vi "CalculerPolynome.vi"(6 "Résidu [in]":dbl, 8 "e3 [in]":dbl, 9 "Meilleure poly [in]":dbl[](array[numeric]), 10 "Y":dbl[](array[numeric]), 11 "X":dbl[](array[numeric])) -> (2 "Résidu [out]":dbl, 3 "Meilleur poly [out]":dbl[](array[numeric]))   [LabVIEW 2013]
uses:
  lm64.dll
  lm32.dll
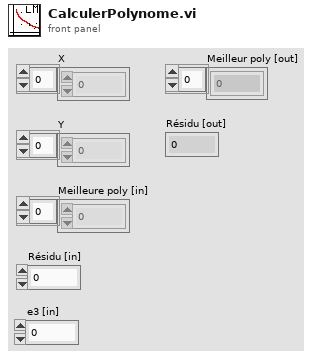
[diagram p1: front panel]
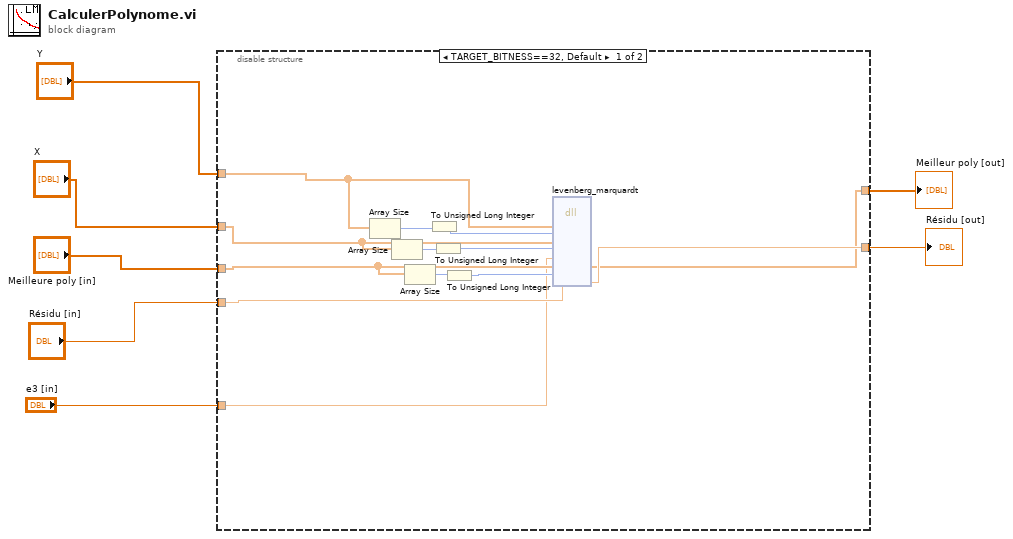
[diagram p0: block diagram]
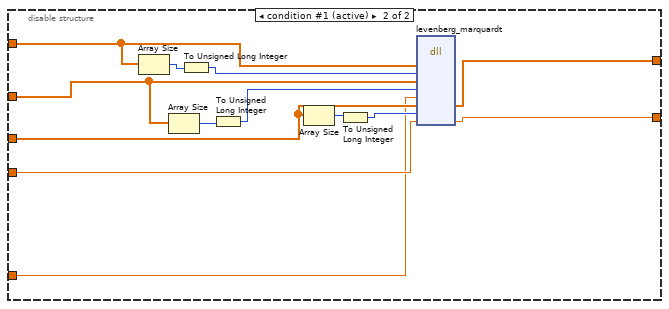
[diagram p2: hidden frame]
diagram:
  n1 = disable-structure shown="TARGET_BITNESS==32, Default" {
    disable-tunnel: "X" -> [w11 w33]
    disable-tunnel: "Y" -> [w14 w32]
    disable-tunnel: "Meilleure poly [in]" -> [w17 w27]
    disable-tunnel: "Résidu [in]" -> [w20 w24]
    disable-tunnel: [w10 w23] -> w6
    disable-tunnel: [w9 w22] -> w7
    disable-tunnel: "e3 [in]" -> [w8 w21]
    frame condition #0 {
      n2 = Array Size(array=w14) -> (size(s)=w15:i32)
      n3 = Array Size(array=w11) -> (size(s)=w12:i32)
      n4 = Array Size(array=w17) -> (size(s)=w18:i32)
      n5 = To Unsigned Long Integer(number=w15) -> (unsigned 32bit integer=w16:u32)
      n6 = To Unsigned Long Integer(number=w12) -> (unsigned 32bit integer=w13:u32)
      n7 = To Unsigned Long Integer(number=w18) -> (unsigned 32bit integer=w19:u32)
      n8 = dll-call lib="C:/Users/Damien/Documents/GitHub/TopView/lm32.dll" fn="levenberg_marquardt"("yobs"=w14, "yobslength"=w16, "xobs"=w11, "xobslength"=w13, "e3"=w8, "polyptr"=w17, "numCoeffs"=w19, "e"=w20) -> ("polyptr"=w9:dbl[], "e"=w10:dbl)  [unwired: 10 in, 2 out]
    }
    frame condition #1 (active) {
      n9 = Array Size(array=w32) -> (size(s)=w29:i32)
      n10 = Array Size(array=w33) -> (size(s)=w31:i32)
      n11 = To Unsigned Long Integer(number=w29) -> (unsigned 32bit integer=w28:u32)
      n12 = To Unsigned Long Integer(number=w31) -> (unsigned 32bit integer=w30:u32)
      n13 = Array Size(array=w27) -> (size(s)=w26:i32)
      n14 = To Unsigned Long Integer(number=w26) -> (unsigned 32bit integer=w25:u32)
      n15 = dll-call lib="C:/Users/Damien/Documents/GitHub/TopView/lm64.dll" fn="levenberg_marquardt"("yobs"=w32, "yobslength"=w28, "xobs"=w33, "xobslength"=w30, "e3"=w21, "polyptr"=w27, "numCoeffs"=w25, "e"=w24) -> ("polyptr"=w22:dbl[], "e"=w23:dbl)  [unwired: 10 in, 2 out]
    }
  }
  "Meilleur poly [out]" <- w7
  "Résidu [out]" <- w6
